vi "Read Required Keys.vi"(8 "error in (no error)":errorcluster, 11 "Configuration in":refnum<class "Configuration.lvclass">) -> (0 "error out":errorcluster, 2 "Required Keys":string[](array[string]), 3 "Configuration out":refnum<class "Configuration.lvclass">)   [LabVIEW 2023, in "Configuration.lvlib" / "Configuration.lvclass"]
doc: "<b>Read Required Keys</b>\n\nOverride and call parent method for this routine. \nThis routine returns an array of all of the required keys for any instantiated device.\n\n<b>Configuration</b> Keys: \n<b>Class</b> - The name of the descendant class which will define the instance\n<b>Category</b> - The type of class (this is used to create the dynamic loading paths)"
uses:
  Library/Configuration.lvclass
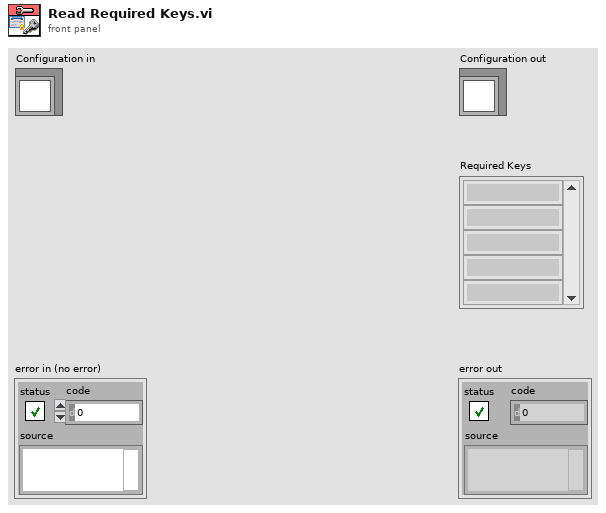
[diagram p1: front panel]
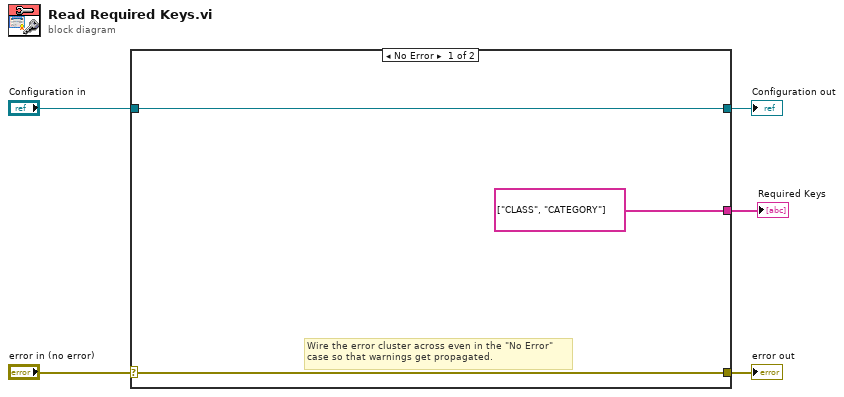
[diagram p0: block diagram]
diagram:
  n1 = case shown="No Error" "error in (no error)" {
    selector: "error in (no error)" -> [w7 w10]
    tunnel: [w7 w10] -> w4
    tunnel: [w8 w9] -> w2
    tunnel: "Configuration in" -> [w8 w9]
    tunnel: [string[] ["CLASS", "CATEGORY"] ("Required Keys") _] -> w1
    frame No Error {
      # "Wire the error cluster across even in the \"No Error\"\ncase so that warnings get propagated."
    }
    frame Error {
    }
  }
  "error out" <- w4
  "Configuration out" <- w2
  "Required Keys" <- w1
